vi "CreateDbCommand.vi"(8 "error in (no error)":errorcluster, 11 "DbConnection in":refnum<class "DbConnection.lvclass">) -> (0 "error out":errorcluster, 2 "CreateCommand":refnum<k24>, 3 "DbConnection out":refnum<class "DbConnection.lvclass">)   [LabVIEW 2020, in "ORM.lvlib" / "DbConnection.lvclass"]
uses:
  DbConnection.lvclass
  System.Data
  DbConnection.lvclass/DbConnection.ctl
  Read connection.vi
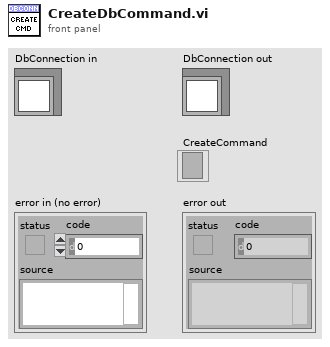
[diagram p1: front panel]
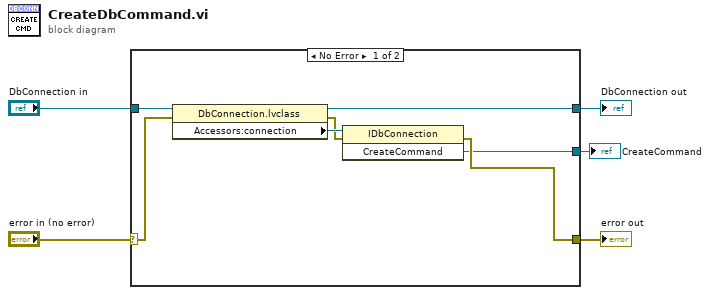
[diagram p0: block diagram]
diagram:
  n1 = case shown="No Error" "error in (no error)" {
    selector: "error in (no error)" -> [w9 w14]
    tunnel: [w7 w14] -> w4
    tunnel: [w10 w13] -> w2
    tunnel: "DbConnection in" -> [w11 w13]
    tunnel: [w6 _] -> w1
    frame No Error {
      n2 = property class="DbConnection.lvclass"(reference=w11, error in=w9) -> (reference out=w10:refnum<class "DbConnection.lvclass">, error out=w8:errorcluster, "Accessors:connection"=w12:refnum<k24>)
      n3 = invoke class="IDbConnection" method="CreateCommand"(reference=w12, error in=w8) -> (error out=w7:errorcluster, "CreateCommand"=w6:refnum<k24>)  [unwired: 1 in, 1 out]
    }
    frame Error {
    }
  }
  "error out" <- w4
  "DbConnection out" <- w2
  "CreateCommand" <- w1
